vi "Oqus RT Driver VI.vi"(7 "Operation":T1, 11 "Device Reference in":T2 format="%.0x") -> (0 "Error Code":i32)   [LabVIEW 2013, in "Oqus Custom Device.lvlib"]
uses:
  Oqus Custom Device.lvlib
  <vilib>/NI Veristand/Custom Device API/Custom Device Item Ref.ctl
  <vilib>/NI Veristand/Custom Device API/Hardware Interface Driver VI Operation.ctl
  <vilib>/NI Veristand/Custom Device API/Custom Device Channel Type.ctl
  <vilib>/NI Veristand/Custom Device API/Data Reference.ctl
  <vilib>/NI Veristand/Custom Device API/Block Data Reference.ctl
  QTMDriver 2013/CustomIO.ctl
  <vilib>/NI Veristand/Custom Device API/Data Access Type.ctl
  <vilib>/NI Veristand/Custom Device API/Global Data Refs.vi
  <vilib>/NI Veristand/Custom Device API/Custom Device API.lvlib
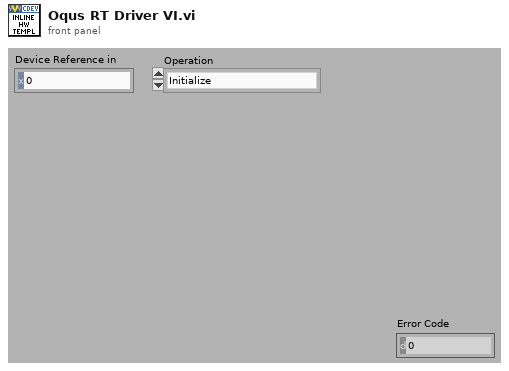
[diagram p1: front panel]
types:
  T1 = typedef "Custom Device API.lvlib/Hardware Interface Driver VI Operation.ctl" = enum16{"Initialize", "Start", "Read Data from HW", "Write Data to HW", "Close"}
  T2 = typedef "Custom Device API.lvlib/Custom Device Item Ref.ctl" = u64
  T3 = typedef "Custom Device API.lvlib/Data Reference.ctl" = i32
  T4 = typedef "Custom Device API.lvlib/Block Data Reference.ctl" = cluster{"Data Reference":T3, "Offset":i32, "Length":i32}
  T5 = cluster{"Input Values":dbl[], "Input Refs":T3[], "Output Values":dbl[], "Output Refs":T3[], "connection ID out":refnum<k5>, "QTMqueue Out":refnum<queue>, "VI Refnum QTMTask Out":refnum<vi>, "Device Error":errorcluster, "InputRefs":T4[], "OutputRefs":T4[]}
  T6 = typedef "Custom Device API.lvlib/Data Access Type.ctl" = enum16{"Read", "Write"}
  T7 = typedef "CustomIO.ctl" = enum16{"Init", "Read", "Write", "Close", "N/O"}
  T8 = typedef "Custom Device API.lvlib/Custom Device Channel Type.ctl" = enum16{"Input", "Output"}
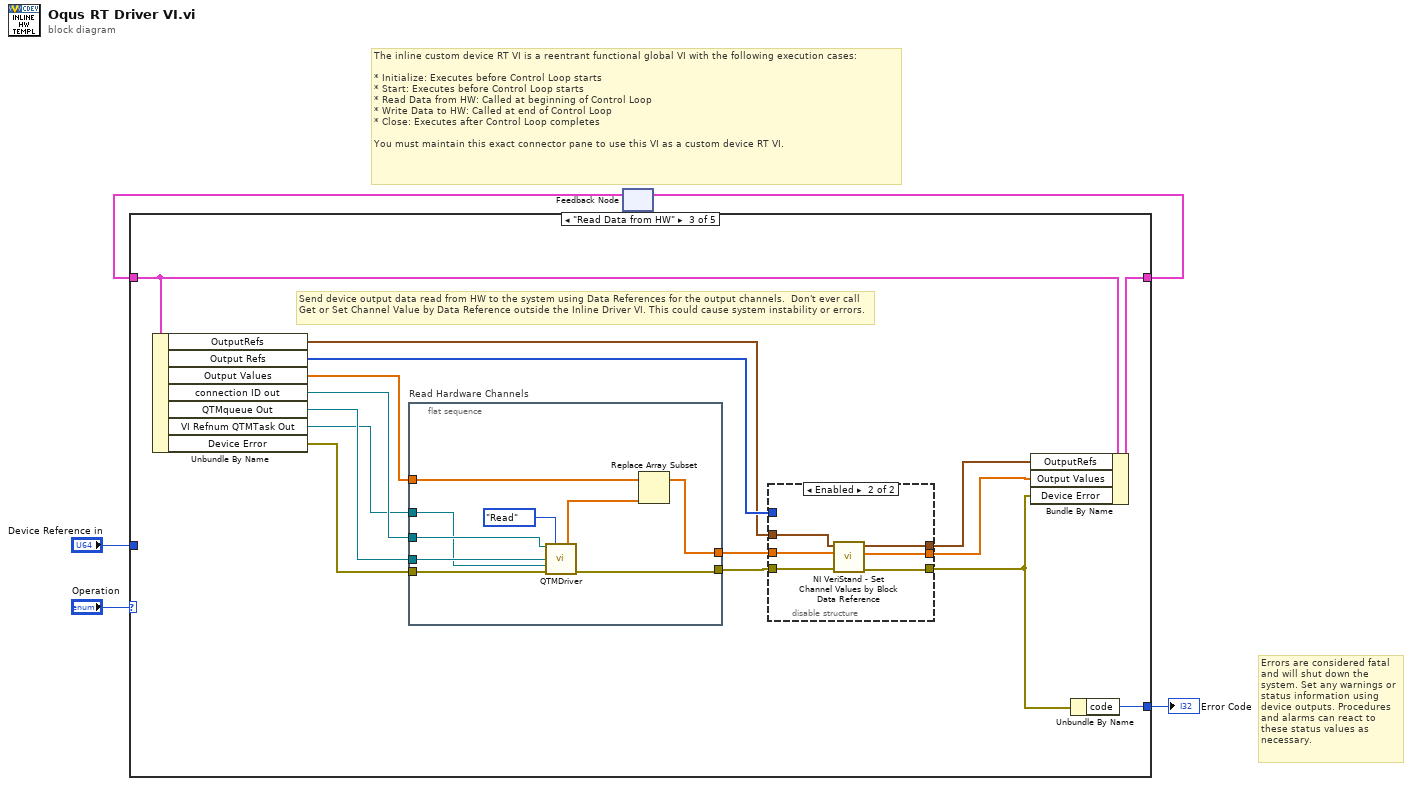
[diagram p0: block diagram]
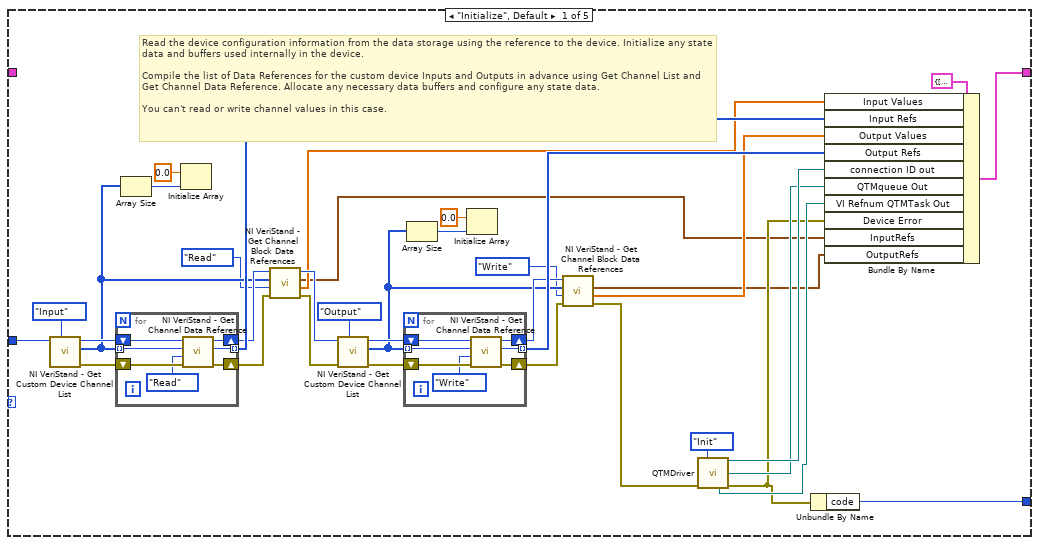
[diagram p2: hidden frame]
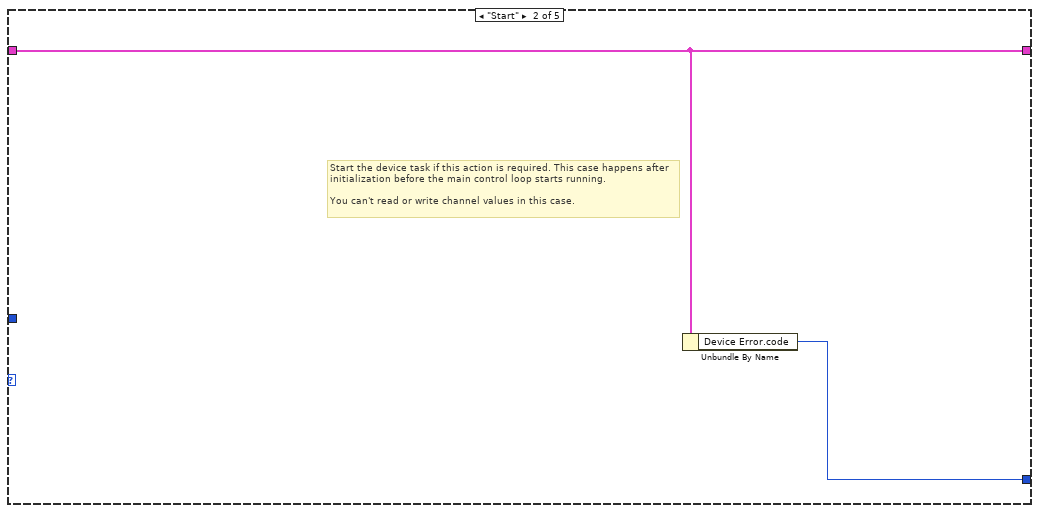
[diagram p3: hidden frame]
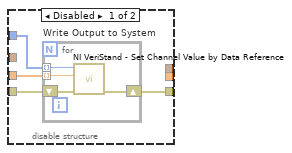
[diagram p4: hidden frame]
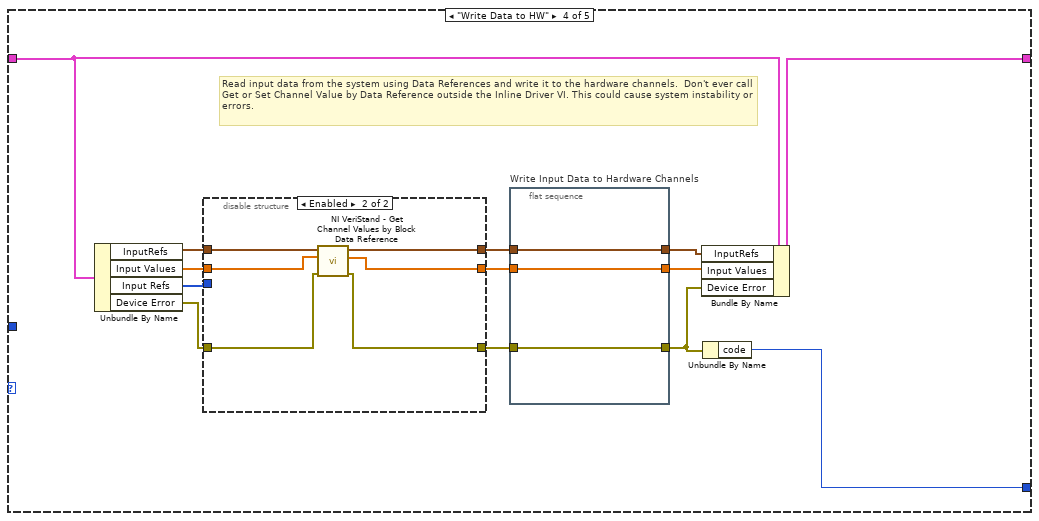
[diagram p5: hidden frame]
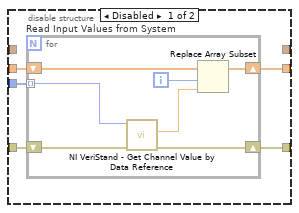
[diagram p6: hidden frame]
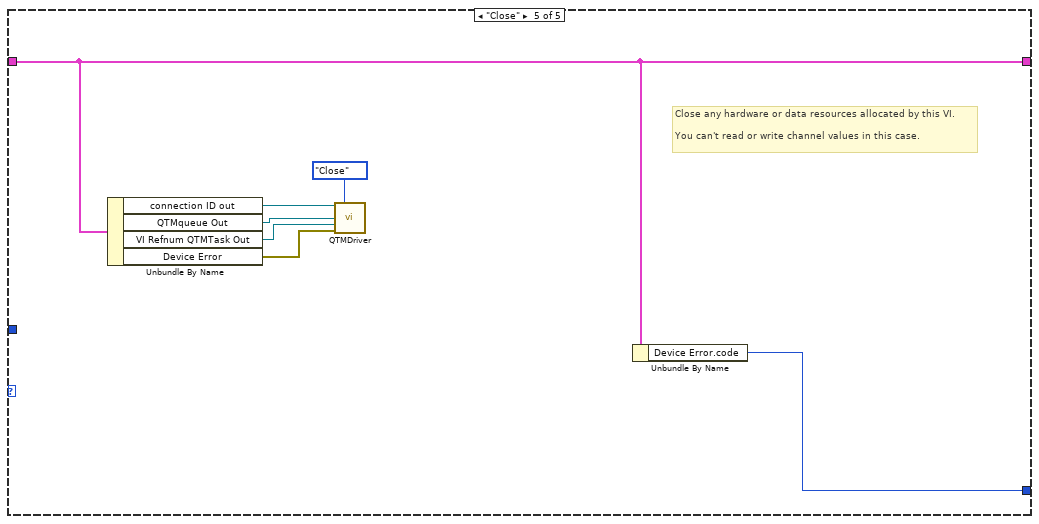
[diagram p7: hidden frame]
diagram:
  # "Errors are considered fatal and will shut down the system. Set any warnings or status information using device outputs. Procedures and alarms can react to these status values as necessary."
  # "The inline custom device RT VI is a reentrant functional global VI with the following execution cases:\n\n* Initialize: Executes before Control Loop starts\n* Start: Executes before Control Loop starts\n* Read Data from HW: Called at beginning of Control Loop\n* Write Data to HW: Called at end of Control Loop\n* Close: Executes after Control Loop completes\n\nYou must maintain this exact connector pane to use this VI as a custom device RT VI."
  n1 = feedback #1() -> (w3:T5)  [unwired: 1 out]
  n2 = case shown="\"Read Data from HW\"" "Operation" {
    tunnel: [w37 w56 w70 w107 w135] -> w4
    tunnel: w3 -> [_ w56 w71 w108 w135]
    tunnel: "Device Reference in" -> [w38 _ _ _ _]
    tunnel: [w36 w57 w61 w105 w136] -> w1
    frame "Initialize", Default {
      # "Read the device configuration information from the data storage using the reference to the device. Initialize any state data and buffers used internally in the device.\n\nCompile the list of Data References for the custom device Inputs and Outputs in advance using Get Channel List and Get Channel Data Reference. Allocate any necessary data buffers and configure any state data.\n\nYou can't read or write channel values in this case."
      n3 = call <vilib>:"NI VeriStand - Get Custom Device Channel List.vi"("Channel Type"=Custom_Device_Channel_Type."Input", "Device Ref in"=w38) -> ("error out"=w34:errorcluster, "Specified Channel Ref List"=w19:T2[], "Device Ref out"=w35:T2)  [unwired: 1 in, 6 out]
      n4 = for {
        shift-right: [w50] -> w21
        shift-left: w35 -> [w54]
        tunnel: w19 -> [w53] mode=indexing
        shift-right: [w51] -> w17
        shift-left: w34 -> [w55]
        tunnel: [w49] -> w30 mode=indexing
        n5 = call <vilib>:"NI VeriStand - Get Channel Data Reference.vi"("error in (no error)"=w55, "Access"=Data_Access_Type."Read", "Channel Ref in"=w53, "Device Ref in"=w54) -> ("error out"=w51:errorcluster, "Channel Data Reference"=w49:T3, "Device Ref out"=w50:T2)  [unwired: 5 out]
      }
      n6 = Array Size(array=w19) -> (size(s)=w41:i32)
      n7 = Initialize Array(0.0 ("element"), w41) -> ()  [unwired: 1 out]
      n8 = call <vilib>:"NI VeriStand - Get Channel Block Data References.vi"("error in (no error)"=w17, "Access"=Data_Access_Type."Read", "Channel Refs"=w19, "Device Ref in"=w21) -> ("error out"=w16:errorcluster, "Values Array"=w15:dbl[], "Block Data Refs"=w7:T4[], "Device Ref out"=w20:T2)  [unwired: 4 in]
      n9 = call <vilib>:"NI VeriStand - Get Custom Device Channel List.vi"("Channel Type"=Custom_Device_Channel_Type."Output", "error in (no error)"=w16, "Device Ref in"=w20) -> ("error out"=w33:errorcluster, "Specified Channel Ref List"=w13:T2[], "Device Ref out"=w32:T2)  [unwired: 6 out]
      n10 = for {
        tunnel: w13 -> [w46] mode=indexing
        shift-right: [w44] -> w11
        shift-left: w33 -> [w48]
        tunnel: [w43] -> w27 mode=indexing
        shift-right: [w42] -> w14
        shift-left: w32 -> [w47]
        n11 = call <vilib>:"NI VeriStand - Get Channel Data Reference.vi"("error in (no error)"=w48, "Access"=Data_Access_Type."Write", "Channel Ref in"=w46, "Device Ref in"=w47) -> ("error out"=w44:errorcluster, "Channel Data Reference"=w43:T3, "Device Ref out"=w42:T2)  [unwired: 5 out]
      }
      n12 = Array Size(array=w13) -> (size(s)=w28:i32)
      n13 = Initialize Array(0.0 ("element"), w28) -> ()  [unwired: 1 out]
      n14 = call <vilib>:"NI VeriStand - Get Channel Block Data References.vi"("error in (no error)"=w11, "Access"=Data_Access_Type."Write", "Channel Refs"=w13, "Device Ref in"=w14) -> ("error out"=w10:errorcluster, "Values Array"=w8:dbl[], "Block Data Refs"=w6:T4[])  [unwired: 4 in, 1 out]
      n15 = call "QTMDriver.vi"("Ring"=CustomIO."Init", "error in"=w10) -> ("connection ID out"=w24:refnum<k5>, "QTMqueue Out"=w23:refnum<queue>, "VI Refnum QTMTask Out"=w22:refnum<vi>, "error out"=w9:errorcluster)  [unwired: 7 in, 3 out]
      n16 = Unbundle By Name(w9) -> ("code"=w36:i32)
      n17 = Bundle By Name(cluster=T5 {"Input Values"=[], "Input Refs"=[], "Output Values"=[], "Output Refs"=[], "connection ID out"=refnum, "QTMqueue Out"=refnum, "VI Refnum QTMTask Out"=refnum, "Device Error"={"status"=FALSE, "code"=0, "source"=""}, "InputRefs"=[], "OutputRefs"=[]}, "Input Values"=w15, "Input Refs"=w30, "Output Values"=w8, "Output Refs"=w27, "connection ID out"=w24, "QTMqueue Out"=w23, "VI Refnum QTMTask Out"=w22, "Device Error"=w9, "InputRefs"=w7, "OutputRefs"=w6) -> (w37:T5)
    }
    frame "Start" {
      # "Start the device task if this action is required. This case happens after initialization before the main control loop starts running.\n\nYou can't read or write channel values in this case."
      n18 = Unbundle By Name(w56) -> ("Device Error.code"=w57:i32)
    }
    frame "Read Data from HW" {
      # "Send device output data read from HW to the system using Data References for the output channels.  Don't ever call Get or Set Channel Value by Data Reference outside the Inline Driver VI. This could cause system instability or errors."
      n19 = Unbundle By Name(w71) -> ("OutputRefs"=w67:T4[], "Output Refs"=w68:T3[], "Output Values"=w72:dbl[], "connection ID out"=w60:refnum<k5>, "QTMqueue Out"=w59:refnum<queue>, "VI Refnum QTMTask Out"=w58:refnum<vi>, "Device Error"=w69:errorcluster)
      n20 = flat-sequence "Read Hardware Channels" {
        tunnel: w69 -> [w92]
        tunnel: [w91] -> w66
        tunnel: [w94] -> w65
        tunnel: w72 -> [w95]
        tunnel: w60 -> [w90]
        tunnel: w59 -> [w89]
        tunnel: w58 -> [w88]
        frame #0 {
          n21 = call "QTMDriver.vi"("connection ID"=w90, "Ring"=CustomIO."Read", "QTMqueue"=w89, "VI Refnum QTMTask"=w88, "error in"=w92) -> ("ArrayOut"=w87:dbl[], "error out"=w91:errorcluster)  [unwired: 4 in, 5 out]
          n22 = Replace Array Subset(array=w95, new element=w87) -> (w94:dbl[])  [unwired: 1 in]
        }
      }
      n23 = disable-structure shown="Enabled" {
        disable-tunnel: w66 -> [w76 w82]
        disable-tunnel: w68 -> [w75 _]
        disable-tunnel: [w74 w86] -> w62
        disable-tunnel: w65 -> [w73 w81]
        disable-tunnel: [_ w85] -> w63
        disable-tunnel: [_ w84] -> w64
        disable-tunnel: w67 -> [_ w83]
        frame Disabled {
          n24 = for "Write Output to System" {
            shift-right: [w79] -> w74
            shift-left: w76 -> [w80]
            tunnel: w73 -> [w78] mode=indexing
            tunnel: w75 -> [w77] mode=indexing
            n25 = call <vilib>:"NI VeriStand - Set Channel Value by Data Reference.vi"("error in (no error)"=w80, "Value"=w78, "Data Reference in"=w77) -> ("error out"=w79:errorcluster)  [unwired: 8 out]
          }
        }
        frame Enabled {
          n26 = call <vilib>:"NI VeriStand - Set Channel Values by Block Data Reference.vi"("error in (no error)"=w82, "Values Array in"=w81, "Block Data Ref"=w83) -> ("error out"=w86:errorcluster, "Values Array out"=w85:dbl[], "Block Data Ref dup"=w84:T4[])  [unwired: 6 in]
        }
      }
      n27 = Bundle By Name(cluster=w71, "OutputRefs"=w64, "Output Values"=w63, "Device Error"=w62) -> (w70:T5)
      n28 = Unbundle By Name(w62) -> ("code"=w61:i32)
    }
    frame "Write Data to HW" {
      # "Read input data from the system using Data References and write it to the hardware channels.  Don't ever call Get or Set Channel Value by Data Reference outside the Inline Driver VI. This could cause system instability or errors."
      n29 = Unbundle By Name(w108) -> ("InputRefs"=w103:T4[], "Input Values"=w102:dbl[], "Input Refs"=w101:T3[], "Device Error"=w100:errorcluster)
      n30 = disable-structure shown="Enabled" {
        disable-tunnel: w101 -> [w113 _]
        disable-tunnel: w102 -> [w112 w124]
        disable-tunnel: [w111 w123] -> w97
        disable-tunnel: [w110 w121] -> w96
        disable-tunnel: w100 -> [w109 w122]
        disable-tunnel: w103 -> [_ w126]
        disable-tunnel: [_ w125] -> w98
        frame Disabled {
          n31 = for "Read Input Values from System" {
            shift-right: [w114] -> w110
            shift-left: w109 -> [w120]
            tunnel: w113 -> [w119] mode=indexing
            shift-right: [w117] -> w111
            shift-left: w112 -> [w118]
            i -> [w116]
            n32 = call <vilib>:"NI VeriStand - Get Channel Value by Data Reference.vi"("error in (no error)"=w120, "Data Reference in"=w119) -> ("error out"=w114:errorcluster, "Value"=w115:dbl)  [unwired: 8 out]
            n33 = Replace Array Subset(array=w118, new element=w115, index=w116) -> (w117:dbl[])
          }
        }
        frame Enabled {
          n34 = call <vilib>:"NI VeriStand - Get Channel Values by Block Data Reference.vi"("error in (no error)"=w122, "Values Array in"=w124, "Block Data Ref"=w126) -> ("error out"=w121:errorcluster, "Values Array out"=w123:dbl[], "Block Data Ref dup"=w125:T4[])  [unwired: 6 in]
        }
      }
      n35 = flat-sequence "Write Input Data to Hardware Channels" {
        tunnel: w97 -> [w129]
        tunnel: [w129] -> w106
        tunnel: [w128] -> w104
        tunnel: w96 -> [w128]
        tunnel: [w127] -> w99
        tunnel: w98 -> [w127]
        frame #0 {
        }
      }
      n36 = Bundle By Name(cluster=w108, "InputRefs"=w99, "Input Values"=w106, "Device Error"=w104) -> (w107:T5)
      n37 = Unbundle By Name(w104) -> ("code"=w105:i32)
    }
    frame "Close" {
      # "Close any hardware or data resources allocated by this VI.\n\nYou can't read or write channel values in this case."
      n38 = Unbundle By Name(w135) -> ("connection ID out"=w133:refnum<k5>, "QTMqueue Out"=w132:refnum<queue>, "VI Refnum QTMTask Out"=w131:refnum<vi>, "Device Error"=w130:errorcluster)
      n39 = call "QTMDriver.vi"("connection ID"=w133, "Ring"=CustomIO."Close", "QTMqueue"=w132, "VI Refnum QTMTask"=w131, "error in"=w130) -> ()  [unwired: 4 in, 7 out]
      n40 = Unbundle By Name(w135) -> ("Device Error.code"=w136:i32)
    }
  }
  "Error Code" <- w1
  n41 = feedback-in #1(w4) -> ()
